vi "Get Resource ID.vi"(11 "SPI in":refnum<class "SPI.lvclass">) -> (2 "Resource ID":string)   [LabVIEW 2020, in "CTI.lvlib" / "SPI.lvclass"]
uses:
  SPI.lvclass
  SPI.lvclass/SPI.ctl
  GPIO/GPIO.lvclass
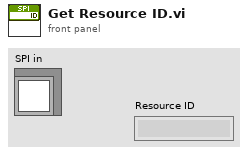
[diagram p1: front panel]
types:
  T1 = typedef "CTI.lvlib/SPI Number.ctl" = i8
  T2 = typedef "CTI.lvlib/GPIO Number.ctl" = i8
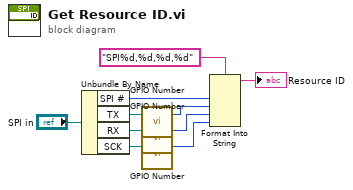
[diagram p0: block diagram]
diagram:
  n1 = Unbundle By Name("SPI in") -> ("SPI #"=w8:T1, "TX"=w6:refnum<class "GPIO.lvclass">, "RX"=w5:refnum<class "GPIO.lvclass">, "SCK"=w4:refnum<class "GPIO.lvclass">)
  n2 = call "GPIO Number.vi"("GPIO in"=w6) -> ("GPIO #"=w3:T2)  [unwired: 6 in]
  n3 = call "GPIO Number.vi"("GPIO in"=w5) -> ("GPIO #"=w2:T2)  [unwired: 6 in]
  n4 = call "GPIO Number.vi"("GPIO in"=w4) -> ("GPIO #"=w1:T2)  [unwired: 6 in]
  n5 = Format Into String(format string="SPI%d,%d,%d,%d", w8, w3, w2, w1) -> (resulting string=→"Resource ID":string)  [unwired: 2 in, 1 out]
